vi "IPI_Cal_XYToCCD_Distance.vi"(8 "error in (no error)":errorcluster, 9 "XY R":dbl=1.0, 10 "Matches (Pattern Matching 1)":T2(array[cluster]) {"Bounding Box"."y" format="%.2f"; "Bounding Box"."x" format="%.2f"; "Position"."y" format="%.2f"; "Position"."x" format="%.2f"; "Score" format="%.2f"; "Scale" format="%.2f"; "Angle" format="%.2f"}, 11 "Image In":T3(plugin-control)) -> (0 "error out":errorcluster, 1 "Y Distance":dbl, 2 "X Distance":dbl, 3 "Image Out":T3(plugin-control))   [LabVIEW 2015]
uses:
  <userlib>/GT400/GT400.lvlib
panel:
  in  "Axis Radio":T1
  out "Y pos":i32
  out "X pos":i32
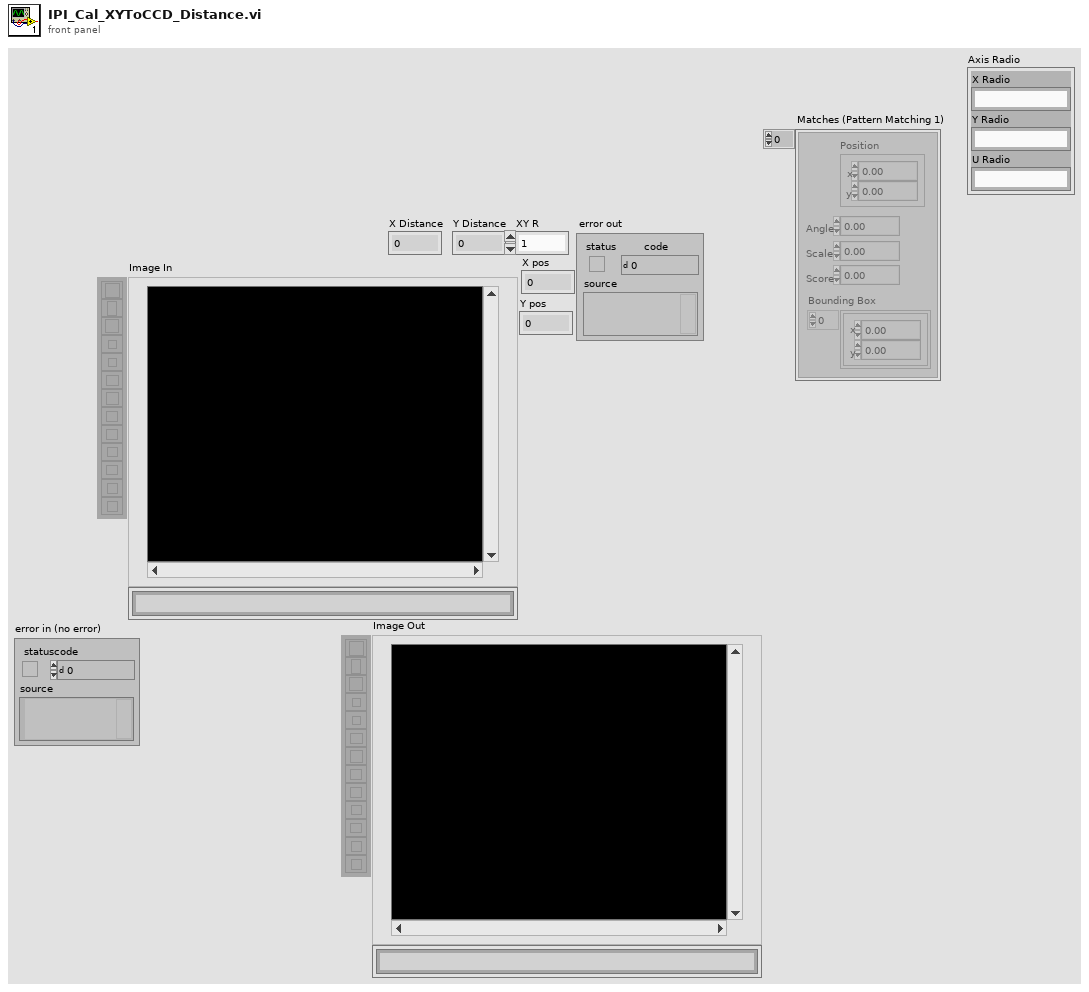
[diagram p1: front panel]
types:
  T1 = cluster{"X Radio":string, "Y Radio":string, "U Radio":string}
  T2 = cluster{"Position":cluster{"x":sgl, "y":sgl}, "Angle":sgl, "Scale":sgl, "Score":sgl, "Bounding Box":cluster{"x":sgl, "y":sgl}[]}[]
  T3 = typedef "IMAQ Image.ctl" = refnum<image>
  T4 = cluster{"Position":cluster{"x":sgl, "y":sgl}, "Angle":sgl, "Scale":sgl, "Score":sgl, "Bounding Box":cluster{"x":sgl, "y":sgl}[]}
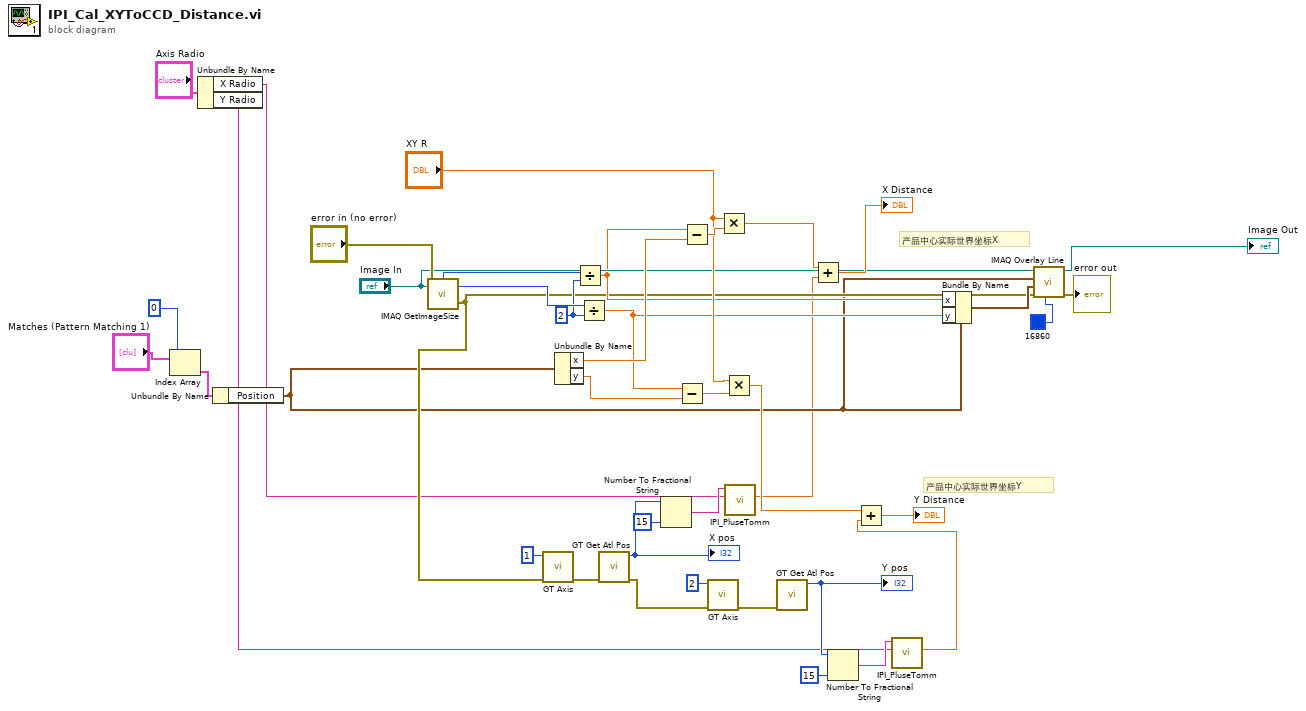
[diagram p0: block diagram]
diagram:
  w39 = 2 ("y")
  # "产品中心实际世界坐标Y"
  # "产品中心实际世界坐标X"
  n1 = Index Array(array="Matches (Pattern Matching 1)", index=0 ("索引")) -> (element=w13:T4)
  n2 = Unbundle By Name("Axis Radio") -> ("X Radio"=w7:string, "Y Radio"=w3:string)
  n3 = Unbundle By Name(w13) -> ("Position"=w12:cluster{"x":sgl, "y":sgl})
  n4 = call "IMAQ GetImageSize"("Image"="Image In", "error in (no error)"="error in (no error)") -> ("Y Resolution"=w40:i32, "X Resolution"=w41:i32, "error out"=w17:errorcluster)  [unwired: 2 in]
  n5 = call <userlib>:"GT Axis.vi"("error in (no error)"=w17, "axis"=u16 1) -> ("error out"=w34:errorcluster)  [unwired: 8 in, 1 out]
  n6 = Unbundle By Name(w12) -> ("x"=w38:sgl, "y"=w37:sgl)
  n7 = Divide(x=w41, y=w39) -> (x/y=w20:dbl)
  n8 = Divide(x=w40, y=w39) -> (x/y=w19:dbl)
  n9 = call <userlib>:"GT Get Atl Pos.vi"("error in (no error)"=w34) -> ("error out"=w31:errorcluster, "pos out"=w10:i32)  [unwired: 8 in, 1 out]
  "X pos" <- w10
  n10 = Number To Fractional String(number=w10, precision (6)=i16 15 ("精度(6)")) -> (F-format string=w8:string)  [unwired: 2 in]
  n11 = Subtract(x=w19, y=w37) -> (x-y=w30:dbl)
  n12 = Subtract(x=w20, y=w38) -> (x-y=w29:dbl)
  n13 = call <userlib>:"GT Axis.vi"("error in (no error)"=w31, "axis"=u16 2) -> ("error out"=w32:errorcluster)  [unwired: 8 in, 1 out]
  n14 = Multiply(x="XY R", y=w29) -> (x*y=w27:dbl)
  n15 = Multiply(x="XY R", y=w30) -> (x*y=w25:dbl)
  n16 = call "IPI_PluseTomm.vi"("Radio"=w7, "Pluse"=w8) -> ("mm"=w2:dbl)  [unwired: 8 in, 1 out]
  n17 = call <userlib>:"GT Get Atl Pos.vi"("error in (no error)"=w32) -> ("pos out"=w4:i32)  [unwired: 8 in, 2 out]
  "Y pos" <- w4
  n18 = Add(x=w27, y=w2) -> (x+y=→"X Distance":dbl)
  n19 = Number To Fractional String(number=w4, precision (6)=i16 15 ("精度(6)")) -> (F-format string=w6:string)  [unwired: 2 in]
  n20 = call "IPI_PluseTomm.vi"("Radio"=w3, "Pluse"=w6) -> ("mm"=w1:dbl)  [unwired: 8 in, 1 out]
  n21 = Add(x=w25, y=w1) -> (x+y=→"Y Distance":dbl)
  n22 = Bundle By Name(cluster=w12, "x"=w20, "y"=w19) -> (w18:cluster{"x":sgl, "y":sgl})
  n23 = call "IMAQ Overlay Line"("Color"=u32 16860, "error in (no error)"=w17, "End Point"=w18, "Start Point"=w12, "Image"="Image In") -> ("error out"=→"error out":errorcluster, "Image Out"=→"Image Out":T3)  [unwired: 5 in]
